vi "Write.vi"(0 "Timeout mS (-1)":i32=-1, 1 "Synchronous (F)":bool, 2 "element":T1, 3 "Close? (F)":bool) -> (5 "Timed Out?":bool, 7 "channel":T2, 8 "Closed?":bool)   [LabVIEW 2022 SP3, in "Flex.lvlib"]
doc: "Updates the shared DVR with the latest value and triggers an occurrence so waiting lossy readers will return the new value. This also writes the value to all active lossless queues.\n\nIf any size limited queues do not have room for the new element within the timeout then the write will be ignored and <b>Timed Out?</b> will return True.\n\nSetting <b>Close?</b> to True will result in all connected reader endpoints reporting the channel as Closed and no further values can be read from the channel.\n\nWhile possible, multiple writer endpoints should not be connected to a single channel. When this is done, as soon as the first writer endpoint sets <b>Close?</b> to true when the entire channel will become invalid."
uses:
  Flex.lvlib
  ))Channel.ctl
  Element.ctl
  ChannelOp.ctl
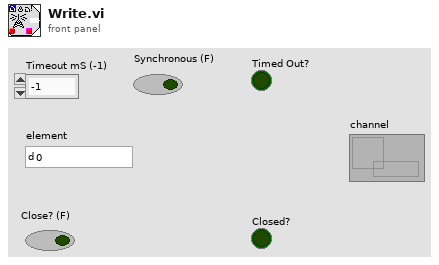
[diagram p1: front panel]
types:
  T1 = typedef "Flex.lvlib/Element.ctl" = dbl
  T2 = typedef "Flex.lvlib/))Channel.ctl" = refnum<queue>
  T3 = typedef "Flex.lvlib/ChannelOp.ctl" = enum16{"Get Refs", "Init", "Close", "Probe", "New Queue", "Remove Queue", "New Event"}
  T4 = typedef "Flex.lvlib/Channel Data.ctl" = cluster{"Element":refnum<data-value>, "Update":refnum<k4>, "Queue Refs":refnum<data-value>, "Event":refnum<user-event>}
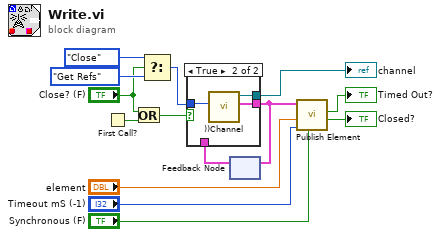
[diagram p0: block diagram]
diagram:
  n1 = First Call?() -> (First Call?: T/F=w10:bool)
  n2 = Or(x="Close? (F)", y=w10) -> (x .or. y?=w11:bool)
  n3 = Select(t=ChannelOp."Close" ("channelOp"), s="Close? (F)", f=ChannelOp."Get Refs" ("channelOp")) -> (s? t:f=w9:T3)
  n4 = feedback #1() -> (w14:T4)  [unwired: 1 in]
  n5 = case shown="True" w11 {
    tunnel: w9 -> [_ w18]
    tunnel: w14 -> [w15 _]
    tunnel: [w15 w16] -> w7
    tunnel: [_ w17] -> w2
    frame False {
    }
    frame True {
      n6 = call "))Channel.vi"("channelOp"=w18) -> ("Channel Data"=w16:T4, "channel out"=w17:T2)  [unwired: 6 in, 3 out]
    }
  }
  "channel" <- w2
  n7 = feedback-in #1(w7) -> ()
  n8 = call "Publish Element.vi"("Synchronous"="Synchronous (F)", "Timeout mS (-1)"="Timeout mS (-1)", "element"="element", "Channel Data In"=w7) -> ("Closed"=→"Closed?":bool, "Timeout"=→"Timed Out?":bool)  [unwired: 6 in]
